vi "Log Init.vi"(6 "Configuration":T1={"Accelerometer Bias"={"X (m/s)"=0.0, "Y (m/s)"=0.0, "Z (m/s)"=0.0}, "Gyroscope Bias"={"X (m/s)"=0.0, "Y (m/s)"=0.0, "Z (m/s)"=0.0}, "Steering Motor Gear Ratio"=611.0, "Steering Pully Gear Ratio"=1.0, "Steering Encoder CPR"=500.0, "Steering Motor Max RPM"=4000.0, "Wheelbase (m)"=1.12, "Fork Angle (rad)"=1.3, "Balancing Controller"={"Kp (/s)"=0.0, "Kd (1)"=0.0}, "Max Allowed Steering Angle (rad)"=0.7, "Task Periods"={"Emergency Stop (us)"=0, "IMU (us)"=0, "Steering Motor Encoder (us)"=0, "State Estimator (us)"=0, "Balancing Controller (us)"=0, "GNSS (us)"=0, "Logging (us)"=0, "Drive Motor (us)"=0}, "Drive Motor Gear Ratio"=0.7, "Drive Motor UART Delay (ms)"=10}, 11 "Error In":errorcluster) -> (2 "Log Handle":T2, 3 "Error Out":errorcluster)   [LabVIEW 2021]
uses:
  Log Handle.ctl
  Configuration/Configuration.ctl
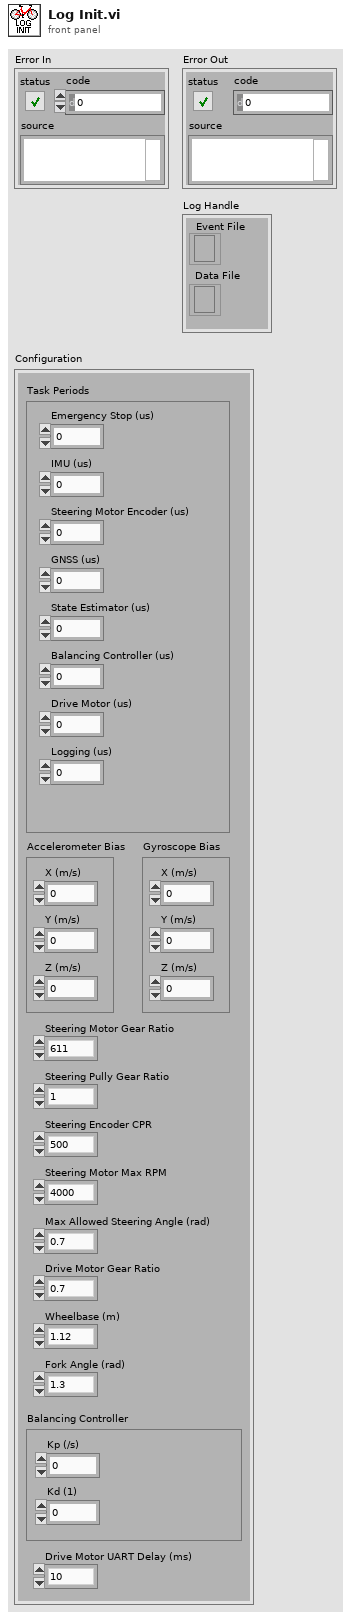
[diagram p1: front panel]
types:
  T1 = typedef "Configuration.ctl" = cluster{"Accelerometer Bias":cluster{"X (m/s)":dbl, "Y (m/s)":dbl, "Z (m/s)":dbl}, "Gyroscope Bias":cluster{"X (m/s)":dbl, "Y (m/s)":dbl, "Z (m/s)":dbl}, "Steering Motor Gear Ratio":dbl, "Steering Pully Gear Ratio":dbl, "Steering Encoder CPR":dbl, "Steering Motor Max RPM":dbl, "Wheelbase (m)":dbl, "Fork Angle (rad)":dbl, "Balancing Controller":cluster{"Kp (/s)":dbl, "Kd (1)":dbl}, "Max Allowed Steering Angle (rad)":dbl, "Task Periods":cluster{"Emergency Stop (us)":i64, "IMU (us)":i64, "Steering Motor Encoder (us)":i64, "State Estimator (us)":i64, "Balancing Controller (us)":i64, "GNSS (us)":i64, "Logging (us)":i64, "Drive Motor (us)":i64}, "Drive Motor Gear Ratio":dbl, "Drive Motor UART Delay (ms)":i64}
  T2 = typedef "Log Handle.ctl" = cluster{"Data File":refnum<file>, "Event File":refnum<file>}
  T3 = enum16{"open", "replace", "create", "open or create", "replace or create", "replace or create with confirmation"}
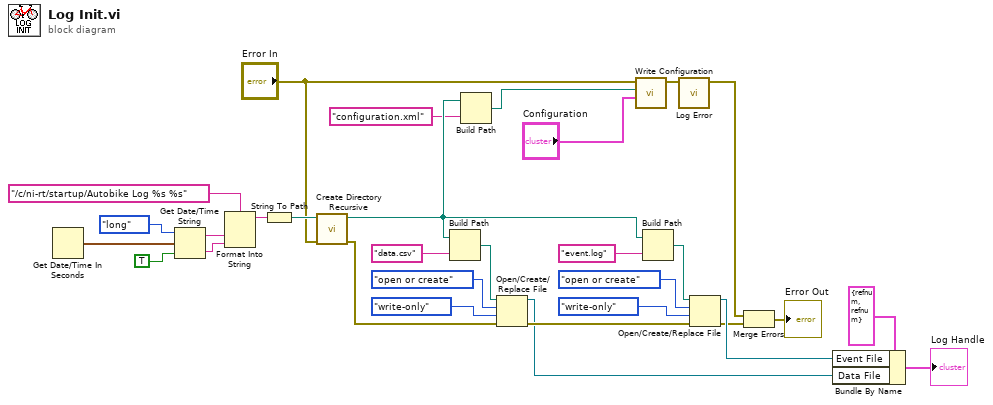
[diagram p0: block diagram]
diagram:
  n1 = Get Date/Time In Seconds() -> (seconds since 1Jan1904=w31:timestamp)
  n2 = Get Date/Time String(date format (0)=enum16{"short", "long", "abbreviated"}."long", seconds (now)=w31, want seconds? (F)=TRUE) -> (date string=w27:string, time string=w26:string)
  n3 = Format Into String(format string="/c/ni-rt/startup/Autobike Log %s %s", w27, w26) -> (resulting string=w23:string)  [unwired: 2 in, 1 out]
  n4 = String To Path(string=w23) -> (path=w20:path)
  n5 = call <vilib>:"Create Directory Recursive.vi"("error in (no error)"="Error In", "directory"=w20) -> ("error out"=w19:errorcluster, "directory copy"=w6:path)  [unwired: 3 in, 1 out]
  n6 = Build Path(base path=w6, name or relative path="data.csv") -> (appended path=w22:path)
  n7 = Build Path(base path=w6, name or relative path="configuration.xml") -> (appended path=w4:path)
  n8 = Open/Create/Replace File(file path (use dialog)=w22, error in=w19, operation (0:open)=T3."open or create", access (0:read/write)=enum16{"read/write", "read-only", "write-only"}."write-only") -> (refnum out=w11:refnum<file>, error out=w12:errorcluster)  [unwired: 2 in, 1 out]
  n9 = call "Write Configuration.vi"("Configuration"="Configuration", "XML File Path"=w4, "Error In"="Error In") -> ("Error Out"=w2:errorcluster)  [unwired: 8 in]
  n10 = Build Path(base path=w6, name or relative path="event.log") -> (appended path=w16:path)
  n11 = call "Log Error.vi"("Error In"=w2) -> ("Error Out"=w1:errorcluster)  [unwired: 10 in]
  n12 = Open/Create/Replace File(file path (use dialog)=w16, error in=w12, operation (0:open)=T3."open or create", access (0:read/write)=enum16{"read/write", "read-only", "write-only"}."write-only") -> (refnum out=w10:refnum<file>, error out=w8:errorcluster)  [unwired: 2 in, 1 out]
  n13 = Merge Errors(w1, w8) -> (→"Error Out":errorcluster)
  n14 = Bundle By Name(cluster=T2 {"Data File"=refnum, "Event File"=refnum} ("Log Handle"), "Event File"=w10, "Data File"=w11) -> (→"Log Handle":T2)
